vi "Simulate.vi"() -> ()   [LabVIEW 2020]
panel:
  out "Matches":i32
  out "Error Out":errorcluster
  in  "Stop":bool
  in  "Inspection Part":enum32{"P2", "P3 Top", "P3 Side"}(tab)
  out "P2 Hole":dbl
  out "P2 Left Edge Angle":dbl
  out "P2 Right Edge Angle":dbl
  out "P2 Hole Status":bool
  out "P2 Left Edge Angle Status":bool
  out "P2 Right Edge Angle Status":bool
  out "P2 Status":bool caption="Status"
  out "P3 Side Top Length":sgl
  out "P3 Hole":dbl
  out "P3 Side Top Length Status":bool
  out "P3 Hole Status":bool
  out "P3 Side Status":bool caption="Status"
  out "Image":T1(plugin-control)
  in  "Start":bool
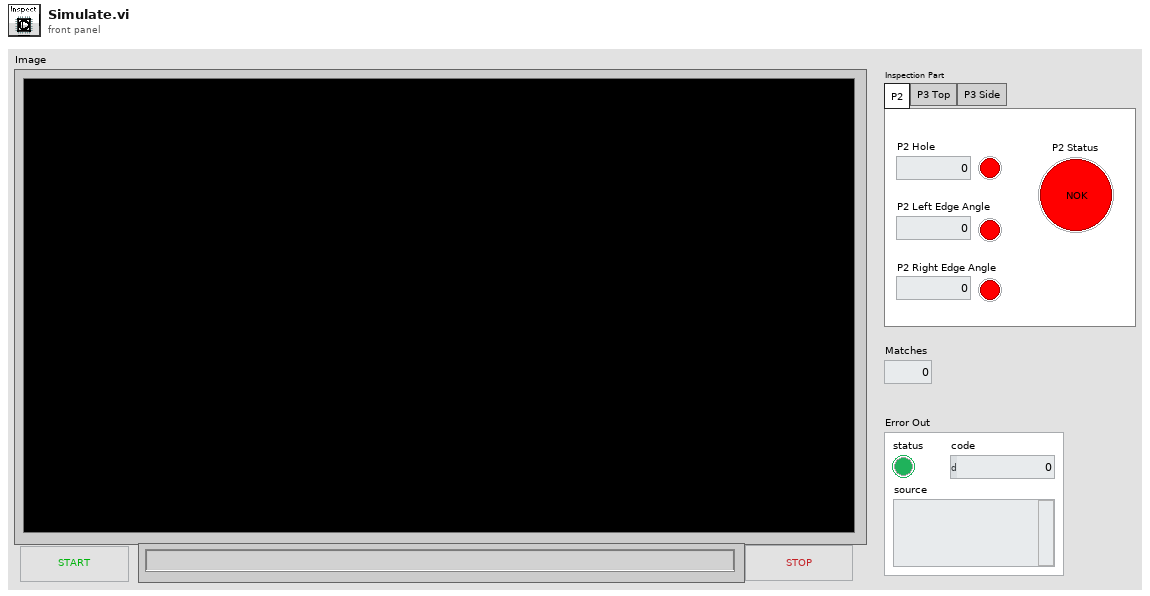
[diagram p1: front panel]
types:
  T1 = typedef "IMAQ Image.ctl" = refnum<image>
  T2 = cluster{"Center (Pixels)":cluster{"X":sgl, "Y":sgl}, "Radius (Pixels)":dbl, "Center (Real-World)":cluster{"X":sgl, "Y":sgl}, "Radius (Real-World)":dbl, "Roundness (Real-World)":dbl, "Average Strength":dbl, "Average SNR (dB)":dbl}
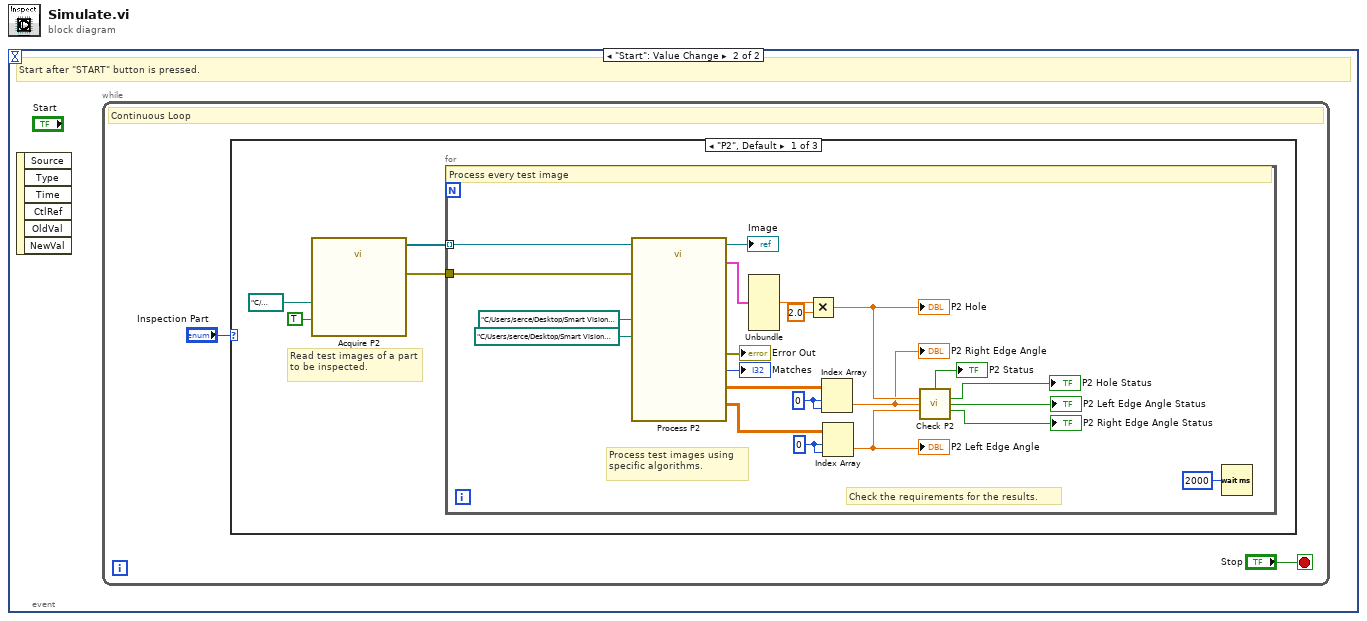
[diagram p0: block diagram]
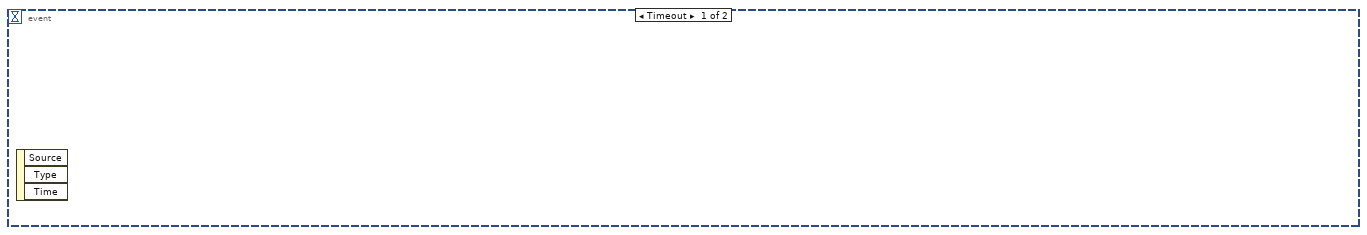
[diagram p2: hidden frame]
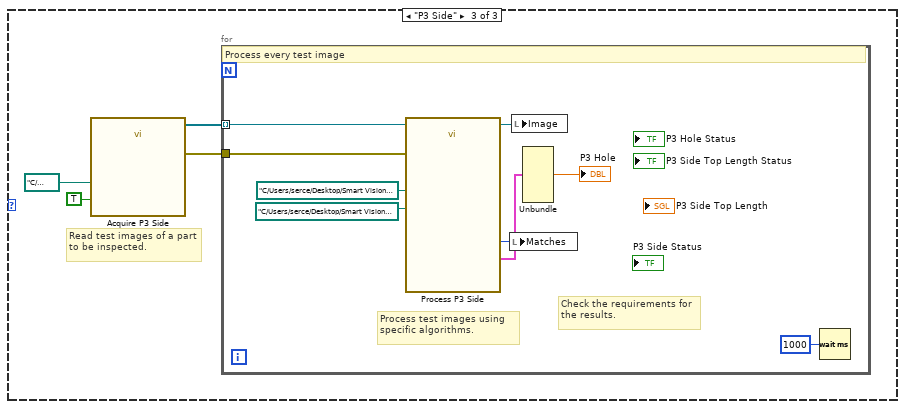
[diagram p4: hidden frame]
diagram:
  n1 = event shown="[1] \"Start\": Value Change" {
    selector: _ -> [_ _]
    dyn-events: _ -> [_ _]
    timeout: _ -> [_ _]
    event Timeout {
      n2 = event-data() -> ()  [unwired: 1 in, 3 out]
    }
    event "Start": Value Change {
      # "Start after \"START\" button is pressed."
      n3 = event-data() -> ()  [unwired: 1 in, 6 out]
      n4 = while {
        stop <- "Stop" stop-if-true
        # "Continuous Loop"
        n5 = case shown="\"P2\", Default" "Inspection Part" {
          frame "P2", Default {
            # "Read test images of a part to be inspected."
            n6 = call "Acquire P2"("Image Path"=path "C:/Users/serce/Desktop/Smart Vision System Testbench/Test Images/P2/P2_0000.png", "Cycle Through Folder"=TRUE) -> ("All Images Out"=w5:T1[], "error out"=w4:errorcluster)  [unwired: 24 in]
            n7 = for {
              tunnel: w5 -> [w24] mode=indexing
              tunnel: w4 -> [w23]
              w16 = 0 ("index (row)")
              w17 = 0 ("index (row)")
              # "Check the requirements for the results."
              # "Process test images using specific algorithms."
              # "Process every test image"
              n8 = call "Process P2"("Image In"=w24, "File Path (Image Calibration P2)"=path "C:/Users/serce/Desktop/Smart Vision System Testbench/Grid Calibration.png" ("Calibration Grid File Path"), "Template File Path (Locate P2 Hole)"=path "C:/Users/serce/Desktop/Smart Vision System Testbench/P2/P2 Hole Template.png" ("Template File Path (P2 Hole)"), "error in"=w23) -> ("Image Out"=→"Image":T1, "Number of Matches (Locate P2 Hole)"=→"Matches":i32, "Fitted Circle (P2 Hole)"=w22:T2, "Calibrated Results (P2 Left Edge Angles)"=w14:sgl[][], "Calibrated Results (P2 Right Edge Angle)"=w15:sgl[][], "error out"=→"Error Out":errorcluster)  [unwired: 18 in]
              n9 = Unbundle(w22) -> ("Radius (Real-World)"=w19:dbl)  [unwired: 6 out]
              n10 = Multiply(x=w19, y=2.0) -> (x*y=w13:dbl)
              "P2 Hole" <- w13
              n11 = Index Array(array=w15, index (row)=w17, index (col)=w17) -> (element=w12:sgl)
              "P2 Right Edge Angle" <- w12
              n12 = Index Array(array=w14, index (row)=w16, index (col)=w16) -> (element=w11:sgl)
              "P2 Left Edge Angle" <- w11
              n13 = call "Check P2.vi"("Calibrated Results (P2 Hole)"=w13, "Calibrated Results (P2 Right Edge Angle)"=w12, "Calibrated Results (P2 Left Edge Angles)"=w11) -> ("P2 Status"=→"P2 Status":bool, "P2 Hole Status"=→"P2 Hole Status":bool, "P2 Left Edge Angle Status"=→"P2 Left Edge Angle Status":bool, "P2 Right Edge Angle Status"=→"P2 Right Edge Angle Status":bool)  [unwired: 9 in]
              n14 = Wait (ms)(milliseconds to wait=u32 2000) -> ()  [unwired: 1 out]
            }
          }
          frame "P3 Top" {
          }
          frame "P3 Side" {
            # "Read test images of a part to be inspected."
            n15 = call "Acquire P3 Side"("Image Path"=path "C:/Users/serce/Desktop/Smart Vision System Testbench/Test Images/P3 Side/P3_Side0000.png", "Cycle Through Folder"=TRUE) -> ("All Images Out"=w31:T1[], "error out"=w30:errorcluster)  [unwired: 24 in]
            n16 = for {
              tunnel: w31 -> [w41] mode=indexing
              tunnel: w30 -> [w40]
              # "Check the requirements for the results."
              # "Process test images using specific algorithms."
              # "Process every test image"
              n17 = call "Process P3 Side"("Image In"=w41, "File Path (Calibrate Grid P3)"=path "C:/Users/serce/Desktop/Smart Vision System Testbench/Grid Calibration.png", "Template File Path (Locate P3 Corner)"=path "C:/Users/serce/Desktop/Smart Vision System Testbench/P3 Side/P3 Side Template.png", "error in"=w40) -> ("Image Out"=w37:T1, "Number of Matches (Locate P3 Corner)"=w38:i32, "Fitted Circle (P3 Hole)"=w33:T2)  [unwired: 19 in, 2 out]
              n18 = local write "Matches"(w38) -> ()
              n19 = local write "Image"(w37) -> ()
              n20 = Unbundle(w33) -> ("Radius (Real-World)"=→"P3 Hole":dbl)  [unwired: 6 out]
              n21 = Wait (ms)(milliseconds to wait=u32 1000) -> ()  [unwired: 1 out]
            }
          }
        }
      }
    }
  }
